vi "Convert Remote to GUI Events.vi"(4 "Data":T2, 5 "Node Name":string, 6 "Node Color":u32(colorbox)) -> (7 "GUI Events":T1[](array[typedef]))   [LabVIEW 2020, in "Volatus.lvlib" / "Event Reporter Module.lvclass"]
uses:
  Event Reporter Module.lvclass
  Event Reporter Module.lvclass/Event Reporter Module.ctl
  Event Element.ctl
  lv-vecto/Vecto/Vecto.lvlib
  Event Level.ctl
  Volatus.lvlib
  messages/Error/Data.ctl
  messages/Error/Error.lvlib
  messages/EventLevel/Enumeration.ctl
  messages/EventLevel/EventLevel.lvlib
  messages/Event/Data.ctl
  messages/Event/Event.lvlib
  messages/Events/Data.ctl
  messages/Events/Events.lvlib
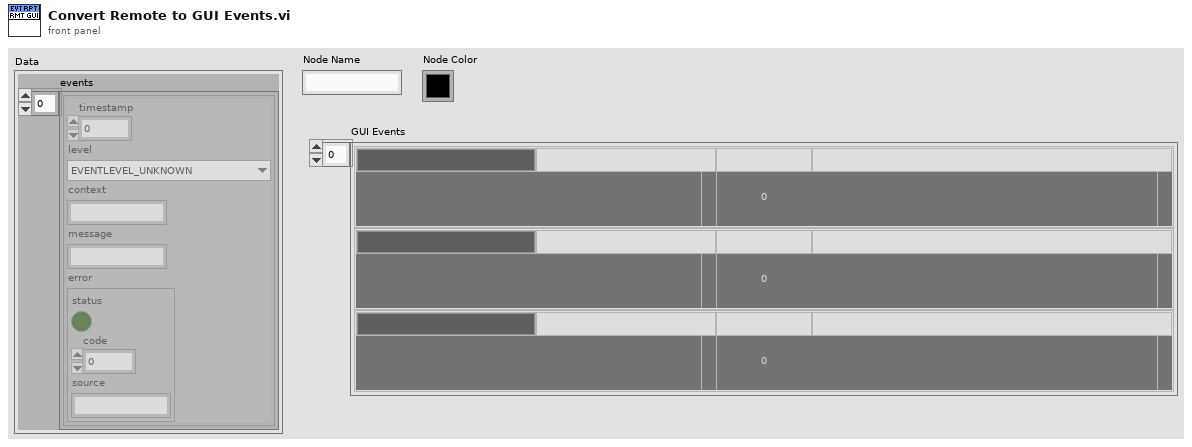
[diagram p1: front panel]
types:
  T1 = typedef "Volatus.lvlib/Event Reporter Module.lvclass/Event Element.ctl" = cluster{"Node":string, "Node Color":u32, "Timestamp":string, "TS Color":u32, "Level":string, "Level Color":u32, "Context":string, "Context Color":u32, "Message":string, "Error Code":i32, "Error Source":string}
  T2 = typedef "Events.lvlib/Data.ctl" = cluster{"events":T3[]}
  T3 = typedef "Event.lvlib/Data.ctl" = cluster{"timestamp":i64, "level":T4, "context":string, "message":string, "error":T5}
  T4 = typedef "EventLevel.lvlib/Enumeration.ctl" = enum16{"EVENTLEVEL_UNKNOWN", "EVENTLEVEL_DEBUG", "EVENTLEVEL_INFO", "EVENTLEVEL_WARNING", "EVENTLEVEL_ERROR"}
  T5 = typedef "Error.lvlib/Data.ctl" = errorcluster
  T6 = typedef "Volatus.lvlib/Event Level.ctl" = enum16{"Debug", "Info", "Warning", "Error"}
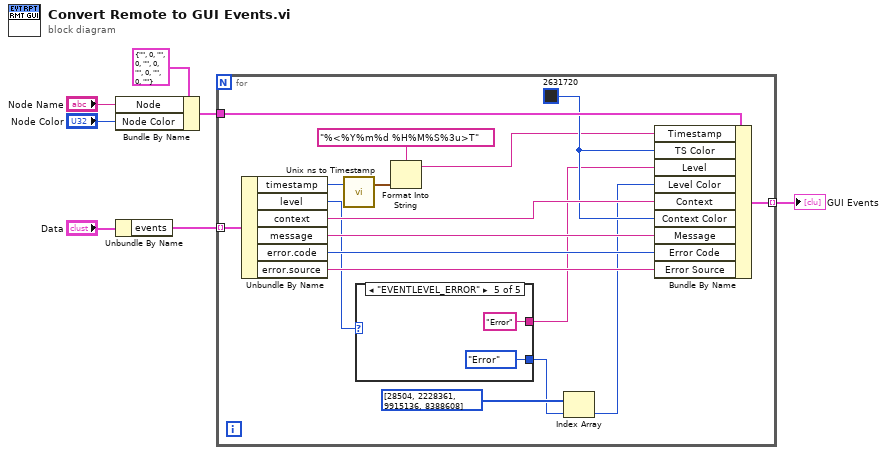
[diagram p0: block diagram]
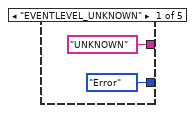
[diagram p2: hidden frame]
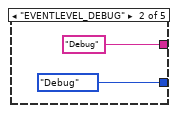
[diagram p3: hidden frame]
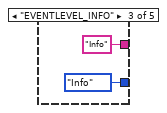
[diagram p4: hidden frame]
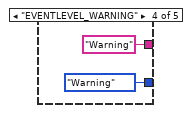
[diagram p5: hidden frame]
diagram:
  n1 = Bundle By Name(cluster=T1 {"Node"="", "Node Color"=0, "Timestamp"="", "TS Color"=0, "Level"="", "Level Color"=0, "Context"="", "Context Color"=0, "Message"="", "Error Code"=0, "Error Source"=""} ("Event Element"), "Node"="Node Name", "Node Color"="Node Color") -> (w2:T1)
  n2 = Unbundle By Name("Data") -> ("events"=w3:T3[])
  n3 = for {
    tunnel: w3 -> [w23] mode=indexing
    tunnel: w2 -> [w24]
    tunnel: [w8] -> w1 mode=indexing
    w18 = u32 2631720 ("Context Color")
    n4 = Unbundle By Name(w23) -> ("timestamp"=w16:i64, "level"=w17:T4, "context"=w19:string, "message"=w20:string, "error.code"=w21:i32, "error.source"=w22:string)
    n5 = call "Unix ns to Timestamp.vi"("Unix ns"=w16) -> ("Time Stamp"=w14:timestamp)  [unwired: 2 in]
    n6 = case shown="\"EVENTLEVEL_ERROR\"" w17 {
      tunnel: [Event_Level."Error" ("Event Level") Event_Level."Debug" ("Event Level") Event_Level."Info" ("Event Level") Event_Level."Warning" ("Event Level") Event_Level."Error" ("Event Level")] -> w10
      tunnel: ["UNKNOWN" "Debug" "Info" "Warning" "Error"] -> w9
      frame "EVENTLEVEL_UNKNOWN" {
      }
      frame "EVENTLEVEL_DEBUG" {
      }
      frame "EVENTLEVEL_INFO" {
      }
      frame "EVENTLEVEL_WARNING" {
      }
      frame "EVENTLEVEL_ERROR" {
      }
    }
    n7 = Format Into String(format string="%<%Y%m%d %H%M%S%3u>T", w14) -> (resulting string=w13:string)  [unwired: 2 in, 1 out]
    n8 = Index Array(array=u32[] [28504, 2228361, 9915136, 8388608], index=w10) -> (element=w11:u32)
    n9 = Bundle By Name(cluster=w24, "Timestamp"=w13, "TS Color"=w18, "Level"=w9, "Level Color"=w11, "Context"=w19, "Context Color"=w18, "Message"=w20, "Error Code"=w21, "Error Source"=w22) -> (w8:T1)
  }
  "GUI Events" <- w1
